vi "Impedance tube v0.6.vi"() -> ()   [LabVIEW 2021]
uses:
  <vilib>/ptbypt/Frequency Domain.llb/Real FFT PtByPt.vi
  <vilib>/express/express analysis/Spectral/Block/exnSpectralBlock spectral measurements RMS poly.vi
  <vilib>/express/express analysis/Spectral/Block/exnSpectralBlock spectral measurements RMS DDT.vi
  <vilib>/express/express arith-compare/Formula/XNode/ExpressFormulaBlockNode.xnode
  <vilib>/express/express analysis/Spectral/XNode/ExpressSpectralMeasurementsBlockNode.xnode
  <vilib>/ptbypt/NI_PtbyPt.lvlib
panel:
  out "number of samples 3":i32=2048
  out "number of samples 2":i32=2048
  out "Reflection Coefficient r":dbl[](graph)
  in  "number of samples":i32=2048
  out "Absorption Coefficient":dbl[](graph)
  out "Waveform Graph 2":dynamicdata(graph)
  out "MIC 2":dynamicdata(graph)
  out "FFT2":dynamicdata(graph)
  out "MIC 2":dbl
  out "FFT1":dynamicdata(graph)
  out "MIC 1":dynamicdata(graph)
  out "MIC 1":dbl
  in  "stop (F)":bool
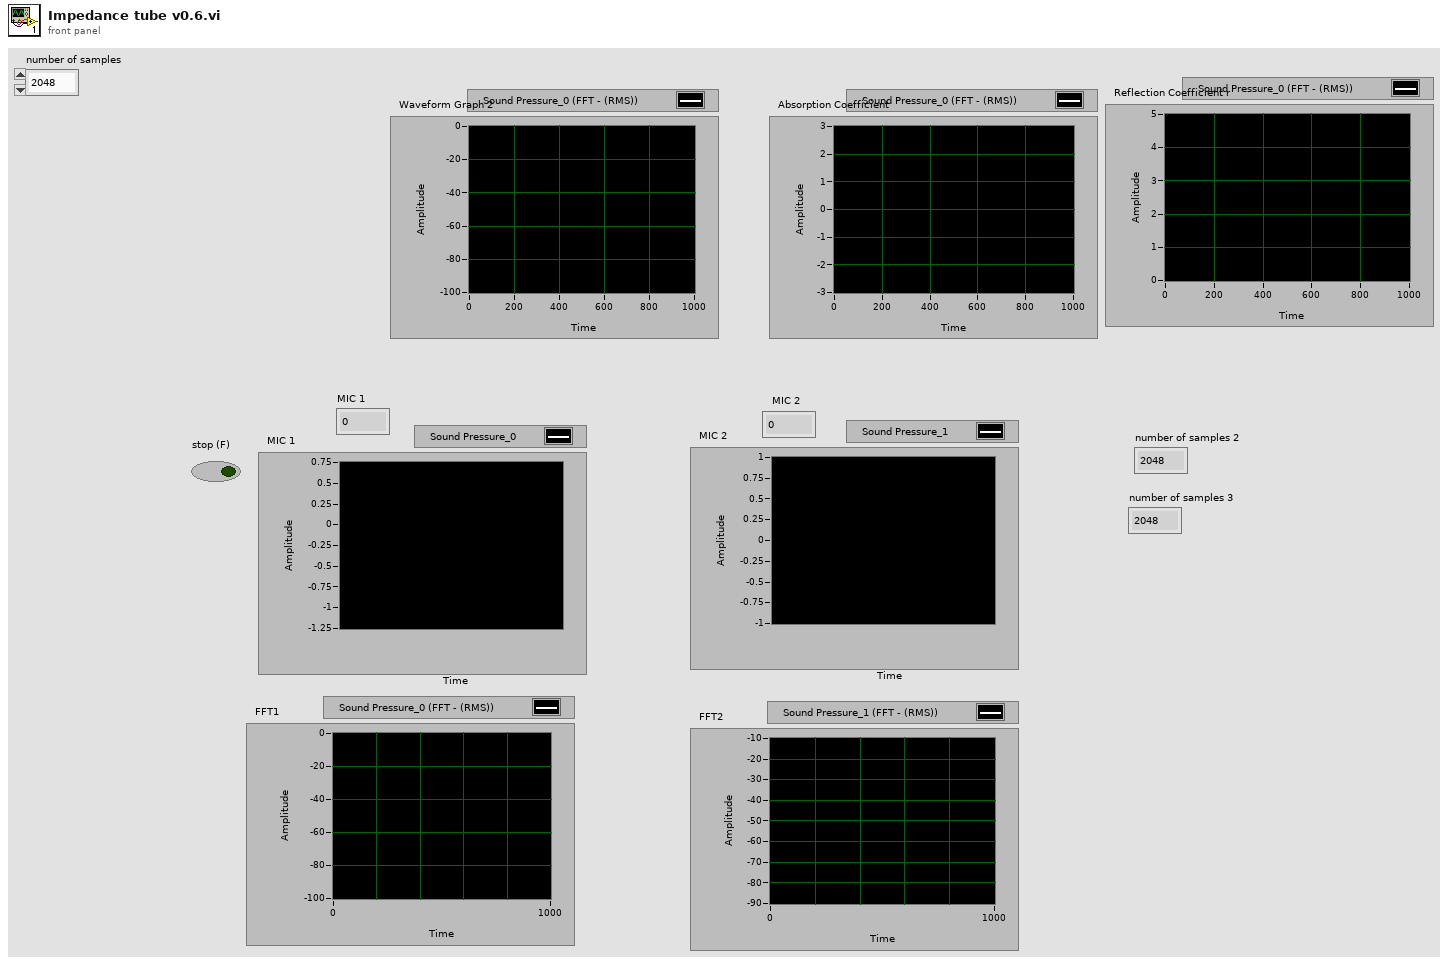
[diagram p1: front panel]
types:
  T1 = cluster{"averaging mode":u16, "weighting mode":u16, "number of averages":u32}
  T2 = cluster{"dB On (F)":bool, "unwrap phase (F)":bool, "convert to degree (F)":bool}
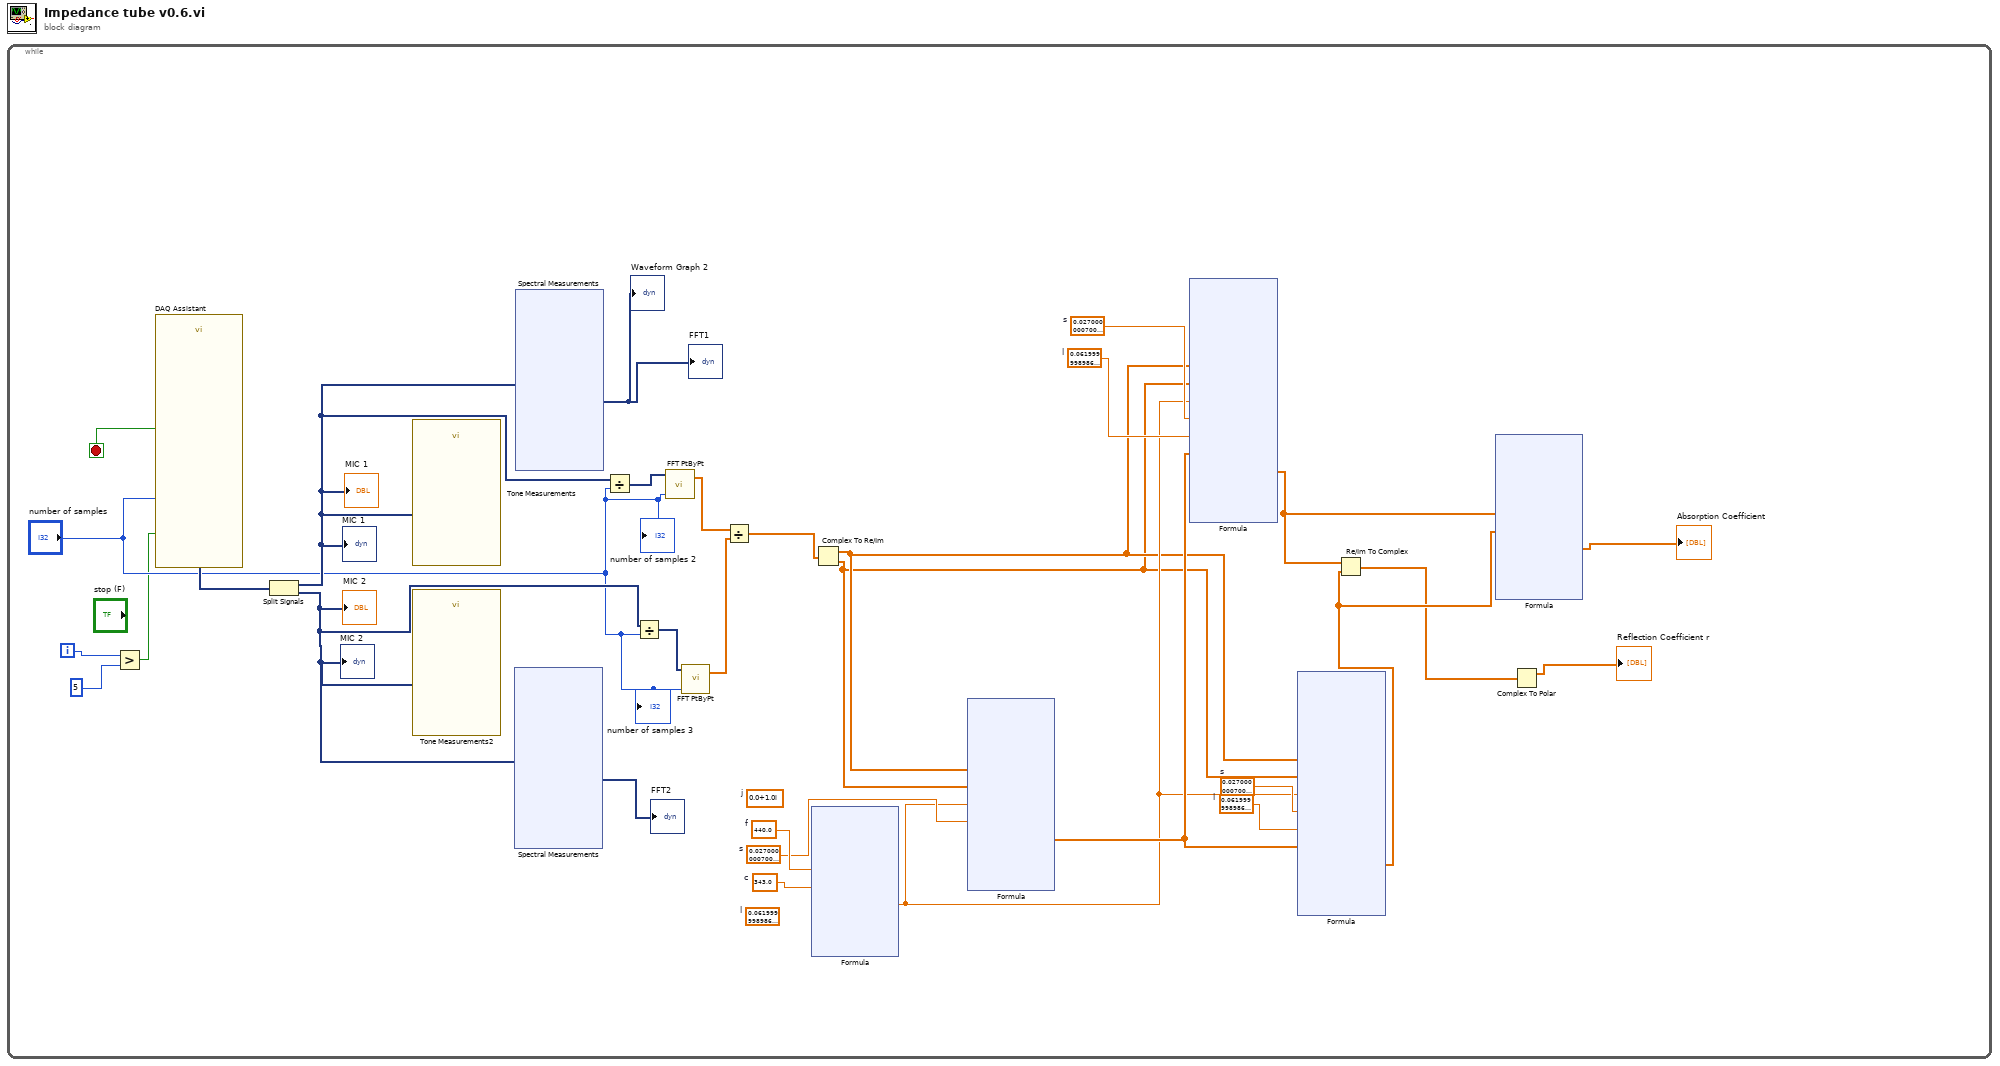
[diagram p0: block diagram]
diagram:
  n1 = while {
    i -> [w3]
    stop <- w31 stop-if-true
    w18 = sgl 0.062  # l
    w19 = sgl 0.027  # s
    w20 = sgl 0.062  # l
    w21 = sgl 0.027  # s
    (unwired) sgl 0.062  # l
    w24 = sgl 440.0  # f
    w22 = sgl 0.027  # s
    w23 = sgl 343.0  # c
    (unwired) csg 0.0+1.0i  # j
    n2 = Greater?(x=w3, y=5) -> (0:w1:bool)
    n3 = call "DAQ Assistant"("number of samples"="number of samples", "stop (F)"=w1) -> ("data"=w30:dynamicdata, "stopped"=w31:bool)  [unwired: 14 in, 2 out]
    n4 = Split Signals(w30) -> (w11:dynamicdata, w9:dynamicdata)  [unwired: 2 in]
    "MIC 1" <- w11
    "MIC 1" <- w11
    "MIC 2" <- w9
    "MIC 2" <- w9
    n5 = call "Tone Measurements"("Signals"=w11) -> ()  [unwired: 8 in, 3 out]
    n6 = call "Tone Measurements2"("Signals"=w9) -> ()  [unwired: 8 in, 3 out]
    n7 = xnode "Spectral Measurements"("Signals"=w9) -> ("FFT - (RMS)"=→"FFT2":dynamicdata)  [unwired: 1 in, 2 out]
    n8 = xnode "Spectral Measurements"("Signals"=w11) -> ("FFT - (RMS)"=→"FFT1" →"Waveform Graph 2":dynamicdata)  [unwired: 1 in, 2 out]
    n9 = Divide(x=w11, y="number of samples") -> (x/y=w10:dynamicdata)
    n10 = Divide(x=w9, y="number of samples") -> (x/y=w8:dynamicdata)
    n11 = call-poly <vilib>:"FFT PtByPt.vi"("sample length"="number of samples", "x"=w10) -> ("FFT{X}"=w25:cdb[])  [unwired: 2 in, 1 out]
    n12 = call-poly <vilib>:"FFT PtByPt.vi"("sample length"="number of samples", "x"=w8) -> ("FFT{X}"=w27:cdb[])  [unwired: 2 in, 1 out]
    n13 = Divide(x=w25, y=w27) -> (x/y=w26:cdb[])
    n14 = xnode "Formula"("f"=w24, "c"=w23) -> ("Result"=w16:sgl)  [unwired: 1 in, 1 out]
    n15 = Complex To Re/Im(x + iy=w26) -> (x=w15:dbl[], y=w14:dbl[])
    n16 = xnode "Formula"("Hr"=w15, "Hi"=w14, "k"=w16, "s"=w22) -> ("Result"=w17:dbl[])  [unwired: 1 in, 1 out]
    n17 = xnode "Formula"("Hr"=w15, "Hi"=w14, "k"=w16, "s"=w21, "l"=w20, "D"=w17) -> ("Result"=w6:dbl[])  [unwired: 1 in, 1 out]
    n18 = xnode "Formula"("Hr"=w15, "Hi"=w14, "k"=w16, "s"=w19, "l"=w18, "D"=w17) -> ("Result"=w13:dbl[])  [unwired: 1 in, 1 out]
    n19 = Re/Im To Complex(1:w13, 2:w6) -> (0:w5:cdb[])
    n20 = xnode "Formula"("Rr"=w6, "Ri"=w13) -> ("Result"=→"Absorption Coefficient":dbl[])  [unwired: 1 in, 1 out]
    n21 = Complex To Polar(r * e^(i*theta)=w5) -> (r=→"Reflection Coefficient r":dbl[])  [unwired: 1 out]
    "number of samples 2" <- "number of samples"
    "number of samples 3" <- "number of samples"
  }
